vi "Piezo_print.vi"(10 "DownStrokeVelocity":dbl, 11 "StrokeLength":dbl) -> (3 ".NET Refnum out":refnum<k24>)   [LabVIEW 2021]
uses:
  C:/Users/csaerome/Documents/PipeJet/PipeJet/Software/bfx_piezo_r13.dll
  Documents/PipeJet/PipeJet/Software/bfx_piezo_r13.dll
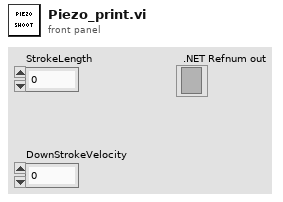
[diagram p1: front panel]
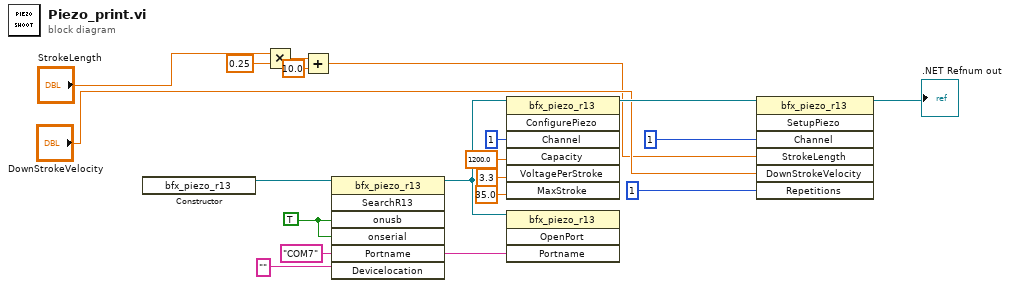
[diagram p0: block diagram]
diagram:
  w18 = TRUE ("onusb")
  n1 = constructor class="bfx_piezo_r13"() -> (reference out=w19:refnum<k24>)  [unwired: 3 in, 2 out]
  n2 = Multiply(x="StrokeLength", y=0.25) -> (x*y=w3:dbl)
  n3 = Add(x=w3, y=10.0) -> (x+y=w1:dbl)
  n4 = invoke class="bfx_piezo_r13" method="SearchR13"(reference=w19, "onusb"=w18, "onserial"=w18, "Portname"="COM7", "Devicelocation"="") -> (reference out=w15:refnum<k24>, "Portname"=w16:string)  [unwired: 2 in, 5 out]
  n5 = invoke class="bfx_piezo_r13" method="ConfigurePiezo"(reference=w15, "Channel"=1, "Capacity"=1200.0, "VoltagePerStroke"=3.3, "MaxStroke"=35.0) -> (reference out=w10:refnum<k24>)  [unwired: 2 in, 6 out]
  n6 = invoke class="bfx_piezo_r13" method="OpenPort"(reference=w15, "Portname"=w16) -> ()  [unwired: 2 in, 4 out]
  n7 = invoke class="bfx_piezo_r13" method="SetupPiezo"(reference=w10, "Channel"=1, "StrokeLength"=w1, "DownStrokeVelocity"="DownStrokeVelocity", "Repetitions"=1) -> (reference out=→".NET Refnum out":refnum<k24>)  [unwired: 2 in, 6 out]
